vi "2_data_type_1.vi"() -> ()   [LabVIEW 2015]
panel:
  out "불리언 2":bool
  in  "불리언":bool
  out "연결된 문자열":string
  out "x+y":dbl
  in  "숫자형 2":dbl
  in  "숫자형":i8
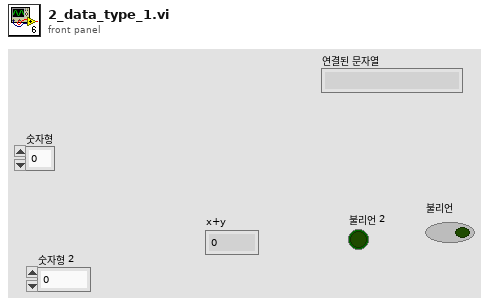
[diagram p1: front panel]
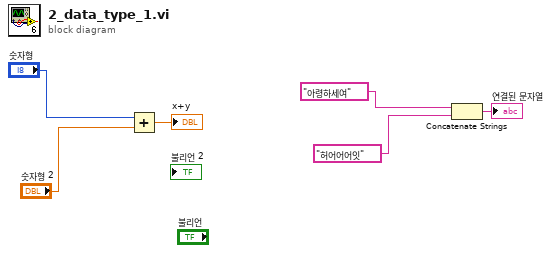
[diagram p0: block diagram]
diagram:
  n1 = Add(x="숫자형", y="숫자형 2") -> (x+y=→"x+y":dbl)
  n2 = Concatenate Strings("아령하세여", "허어어어잇") -> (→"연결된 문자열":string)
